vi "GetSRs.vi"(7 "LabVIEW Web Service Request":refnum<class "Web Request.lvclass">) -> (3 "SRListOut":T1 {"SR#" format="%#_10g"})   [LabVIEW 2017]
uses:
  <vilib>/wsapi/Web Request.lvclass
  ServerLib/TypeDefs/SR List.ctl
  ServerLib/TypeDefs/SR Data.ctl
  ServerLib/SubLibs/WebServiceCommunication/WebServiceFGVcommands.ctl
  ServerLib/SubLibs/WebServiceCommunication/WebServiceCommunication.lvlib
  ServerLib/Server.lvlib
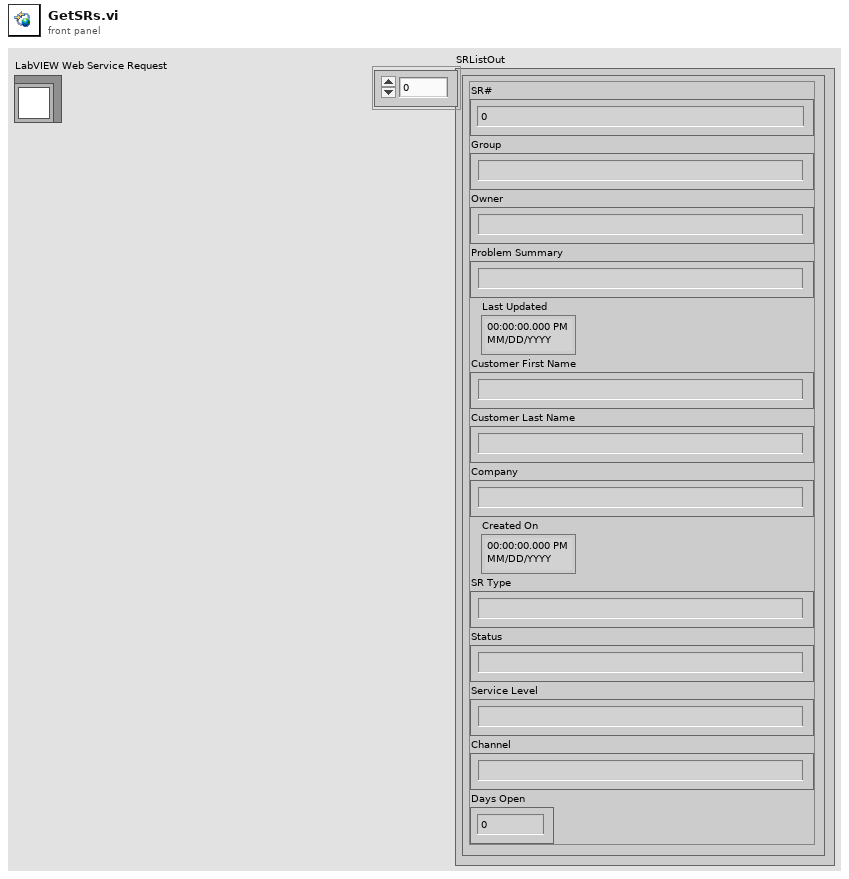
[diagram p1: front panel]
types:
  T1 = typedef "Server.lvlib/SR List.ctl" = T2[]
  T2 = typedef "Server.lvlib/SR Data.ctl" = cluster{"SR#":dbl, "Group":string, "Owner":string, "Problem Summary":string, "Last Updated":timestamp, "Customer First Name":string, "Customer Last Name":string, "Company":string, "Created On":timestamp, "SR Type":string, "Status":string, "Service Level":string, "Channel":string, "Days Open":dbl}
  T3 = typedef "Server.lvlib/WebServiceCommunication.lvlib/WebServiceFGVcommands.ctl" = enum16{"Init", "Reset", "Heartbeat", "GetSRs", "SetSRs", "CheckClients", "GetClients"}
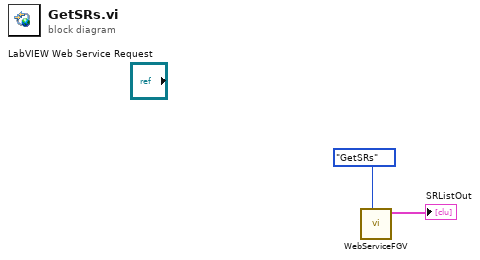
[diagram p0: block diagram]
diagram:
  n1 = call "WebServiceFGV.vi"("CMD"=WebServiceFGVcommands."GetSRs") -> ("SRListOut"=→"SRListOut":T1)  [unwired: 8 in, 2 out]
